vi "magnetometer data without drive coil times in TR.vi"(0 "magnetometer set queue":refnum<queue>, 1 "buffer (s) after":dbl=0.05 format="%#_13g", 2 "t1":dbl=-1.0, 5 "coil":T2, 11 "error in (no error)":errorcluster, 12 "buffer (s) before":dbl=-0.02 format="%#_13g", 13 "t0":dbl=-1.0) -> (4 "mag readings no coil":T1[](array[typedef]), 15 "error out":errorcluster)   [LabVIEW 2017]
uses:
  typedefs/reading queue.ctl
  typedefs/reading.ctl
  typedefs/readingType.ctl
  typedefs/magnetomter reading set.ctl
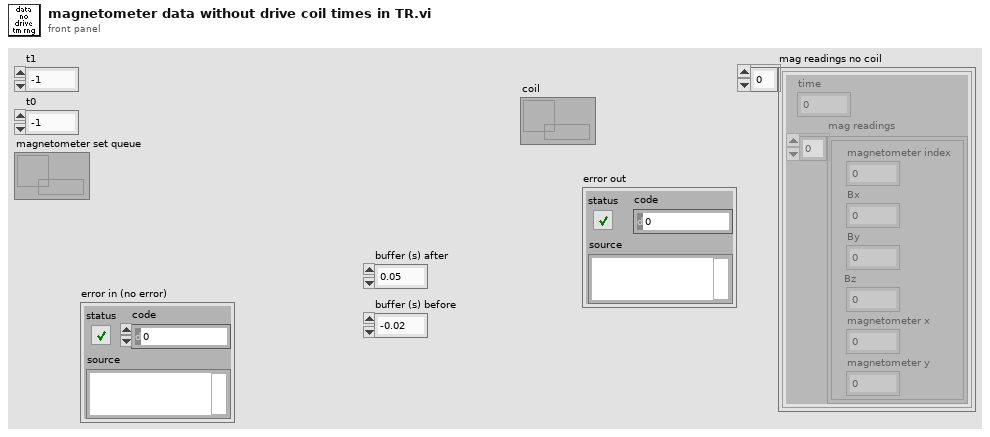
[diagram p1: front panel]
types:
  T1 = typedef "magnetomter reading set.ctl" = cluster{"time":fxp<+,48,48>, "mag readings":cluster{"magnetometer index":dbl, "Bx":dbl, "By":dbl, "Bz":dbl, "magnetometer x":dbl, "magnetometer y":dbl}[]}
  T2 = typedef "reading queue.ctl" = refnum<queue>
  T3 = typedef "reading.ctl" = cluster{"reading type":T4, "time":fxp<+,48,48>, "x":sgl, "y":sgl, "z":sgl, "XSUM":u8}
  T4 = typedef "readingType.ctl" = enum8{"SYNC", "DETVAL", "COILI", "MAGVEC", "ACCVEC", "CROSSING", "MAGVEC0", "MAGVEC1", "MAGVEC2", "MAGVEC3", "MAGVEC4", "MAGVEC5", "MAGVEC6", "MAGVEC7"}
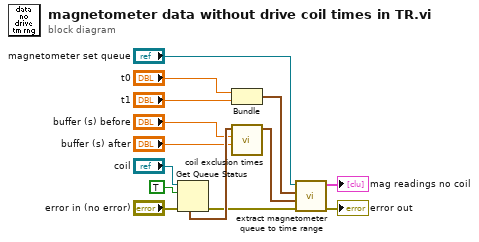
[diagram p0: block diagram]
diagram:
  n1 = Get Queue Status(queue="coil", return elements? (F)=TRUE, error in (no error)="error in (no error)") -> (error out=w3:errorcluster, elements=w11:T3[])  [unwired: 6 out]
  n2 = Bundle("t0"="t0", "t1"="t1") -> (w5:cluster{"t0":dbl, "t1":dbl})  [unwired: 1 in]
  n3 = call "coil exclusion times.vi"("buffer (s) after"="buffer (s) after", "buffer (s) before"="buffer (s) before", "coil elements"=w11) -> ("coil exclusion times"=w8:cluster{dbl, dbl}[])  [unwired: 8 in]
  n4 = call "extract magnetometer queue to time range.vi"("error in (no error)"=w3, "time ranges to exclude"=w8, "time range to include"=w5, "magnetometer set queue"="magnetometer set queue") -> ("error out"=→"error out":errorcluster, "readings in range"=→"mag readings no coil":T1[])  [unwired: 6 in]
